vi "Connect.vi"(8 "error in (no error)":errorcluster, 11 "Postgres Connector In":refnum<class "Postgres Connector.lvclass">) -> (0 "error out":errorcluster, 3 "Postgres Connector Out":refnum<class "Postgres Connector.lvclass">)   [LabVIEW 2019, in "PG_LIB.lvlib" / "Postgres Connector.lvclass"]
doc: "This VI establish a connection with the server using TCP. After, it connect the user to a database."
uses:
  Postgres Connector.lvclass
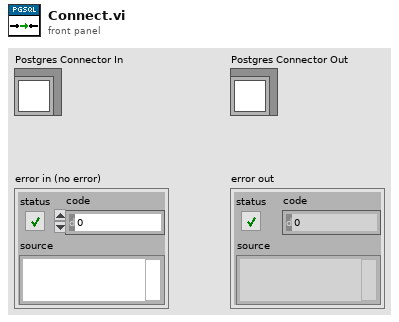
[diagram p1: front panel]
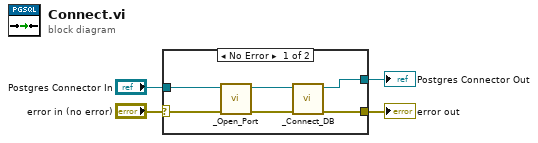
[diagram p0: block diagram]
diagram:
  n1 = case shown="No Error" "error in (no error)" {
    selector: "error in (no error)" -> [w9 w11]
    tunnel: "Postgres Connector In" -> [w10 w12]
    tunnel: [w5 w12] -> w4
    tunnel: [w6 w11] -> w3
    frame No Error {
      n2 = call "_Open_Port.vi"("error in (no error)"=w9, "Postgres Connector.lvclass"=w10) -> ("error out"=w7:errorcluster, "output cluster"=w8:refnum<class "Postgres Connector.lvclass">)  [unwired: 8 in]
      n3 = call "_Connect_DB.vi"("error in (no error)"=w7, "Postgres Connector In"=w8) -> ("error out"=w6:errorcluster, "Postgres Connector Out"=w5:refnum<class "Postgres Connector.lvclass">)  [unwired: 8 in]
    }
    frame Error {
    }
  }
  "error out" <- w3
  "Postgres Connector Out" <- w4
